vi "PXI-Load DO Signal Bank.vi"(4 "error in (no error)":errorcluster, 5 "Input array":bool[][](array[boolean]), 7 "timeout (ms)":i32=5000) -> (0 "error out":errorcluster={"status"=FALSE, "code"=0, "source"="."})   [LabVIEW 2020]
uses:
  Type Defs/PXI-DO Signal Bank Action.ctl
  DAQ Engine VIs/PXI Globals.vi
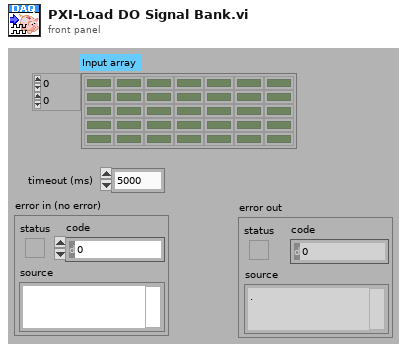
[diagram p1: front panel]
types:
  T1 = typedef "PXI-DO Signal Bank Action.ctl" = enum16{"Clear", "Write", "Read"}
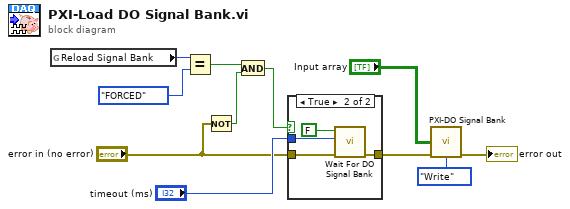
[diagram p0: block diagram]
diagram:
  n1 = global read "PXI Globals.vi" "Reload Signal Bank"() -> (w8:enum32{"OFF", "ENABLED", "FORCED"})
  n2 = Equal?(x=w8, y=enum16{"OFF", "ENABLED", "FORCED"}."FORCED") -> (x = y?=w11:bool)
  n3 = Not(x="error in (no error)") -> (.not. x?=w10:bool)
  n4 = And(x=w11, y=w10) -> (x .and. y?=w7:bool)
  n5 = case shown="True" w7 {
    tunnel: "error in (no error)" -> [w12 w16]
    tunnel: [w12 w14] -> w5
    tunnel: "timeout (ms)" -> [_ w15]
    frame False {
    }
    frame True {
      n6 = call "Wait For DO Signal Bank.vi"("error in (no error)"=w16, "timeout (ms)"=w15, "Desired Fresh State"=FALSE) -> ("error out"=w14:errorcluster)  [unwired: 8 in]
    }
  }
  n7 = call "PXI-DO Signal Bank.vi"("Array"="Input array", "error in (no error)"=w5, "Action"=PXI-DO_Signal_Bank_Action."Write") -> ("error out"=→"error out":errorcluster)  [unwired: 11 in, 1 out]
